vi "OnFrameAvailable_Event_Callback_v2.vi"(4 "User Parameter":T1, 5 "Event Data":cluster{"sender":refnum<k24>, "e":refnum<k24>}, 6 "Control Ref":refnum<k24>, 7 "Event Common Data":T2) -> ()   [LabVIEW 2016]
uses:
  C:/Program Files/Spiricon/BeamSquared/M2.Automation.dll
  M2.Automation.dll
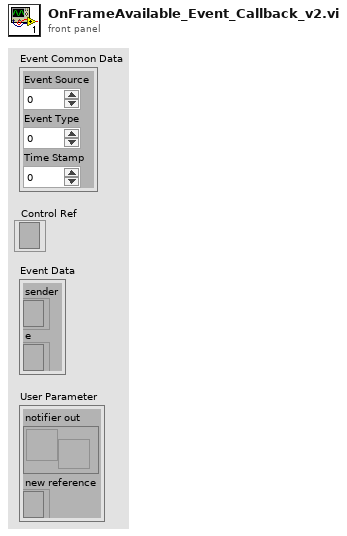
[diagram p1: front panel]
types:
  T1 = cluster{"notifier out":refnum<notifier>, "new reference":refnum<k24>}
  T2 = cluster{"Event Source":i32, "Event Type":u32, "Time Stamp":u32}
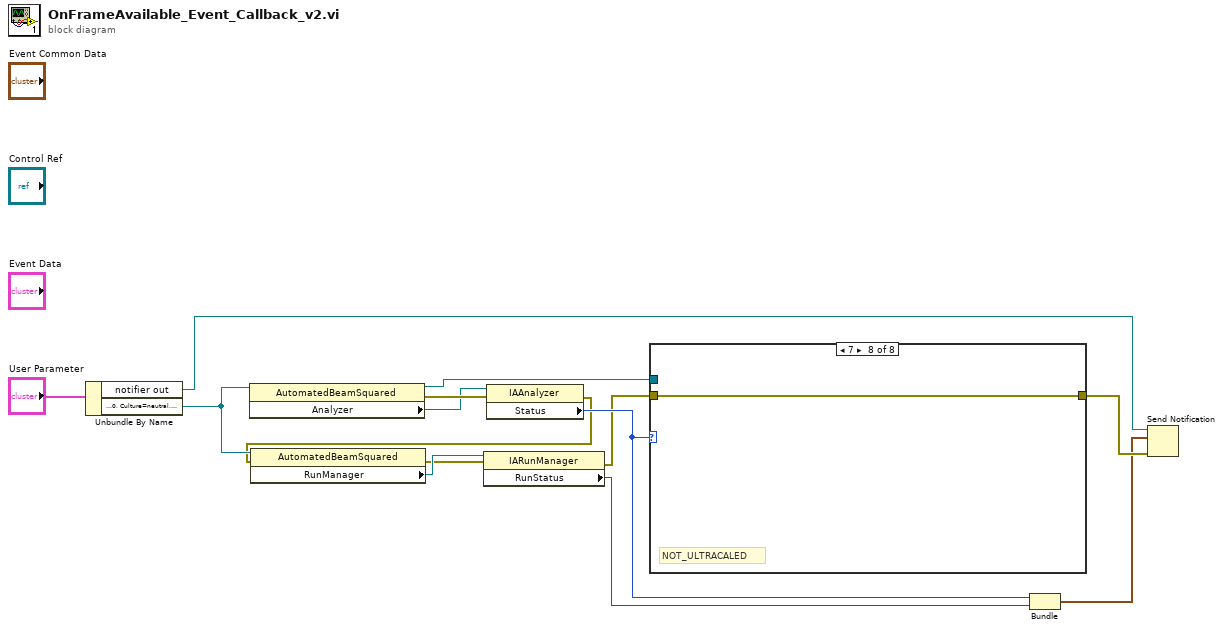
[diagram p0: block diagram]
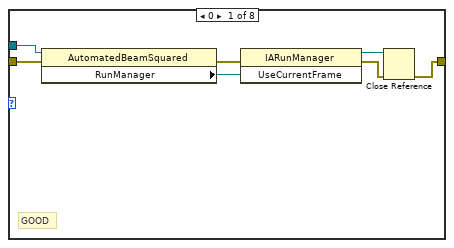
[diagram p2: hidden frame]
diagram:
  n1 = Unbundle By Name("User Parameter") -> ("notifier out"=w14:refnum<notifier>, "new reference"=w6:refnum<k24>)
  n2 = property class="AutomatedBeamSquared"(reference=w6) -> (reference out=w8:refnum<k24>, error out=w13:errorcluster, "Analyzer"=w12:refnum<k24>)  [unwired: 1 in]
  n3 = property class="IAAnalyzer"(reference=w12, error in=w13) -> (error out=w4:errorcluster, "Status"=w9:i32)  [unwired: 1 out]
  n4 = property class="AutomatedBeamSquared"(reference=w6, error in=w4) -> (error out=w5:errorcluster, "RunManager"=w7:refnum<k24>)  [unwired: 1 out]
  n5 = property class="IARunManager"(reference=w7, error in=w5) -> (error out=w3:errorcluster, "RunStatus"=w2:i32)  [unwired: 1 out]
  n6 = case shown="7" w9 {
    tunnel: w3 -> [w21 w22 w23 w24 w25 w26 w27 w28]
    tunnel: [w17 w22 w23 w24 w25 w26 w27 w28] -> w11
    tunnel: w8 -> [w15 _ _ _ _ _ _ _]
    frame 0 {
      # "GOOD"
      n7 = property class="AutomatedBeamSquared"(reference=w15, error in=w21) -> (error out=w20:errorcluster, "RunManager"=w19:refnum<k24>)  [unwired: 1 out]
      n8 = invoke class="IARunManager" method="UseCurrentFrame"(reference=w19, error in=w20) -> (reference out=w18:refnum<k24>, error out=w16:errorcluster)  [unwired: 1 in, 1 out]
      n9 = Close Reference(reference=w18, error in (no error)=w16) -> (error out=w17:errorcluster)
    }
    frame 1, Default {
      # "UNKNOWN"
    }
    frame 2 {
      # "BRIGHT"
    }
    frame 3 {
      # "DIM"
    }
    frame 4 {
      # "BIG"
    }
    frame 5 {
      # "ALIGNMENT"
    }
    frame 6 {
      # "SMALL"
    }
    frame 7 {
      # "NOT_ULTRACALED"
    }
  }
  n10 = Bundle("Status"=w9, "RunStatus"=w2) -> (w10:cluster{"Status":i32, "RunStatus":i32})  [unwired: 1 in]
  n11 = Send Notification(notification=w10, notifier=w14, error in (no error)=w11) -> ()  [unwired: 2 out]
